vi "fpga_Filter Constant.vi"() -> (0 "Total Delay":u8=109, 1 "Start":fxp<+/-,4,4>=1.0, 2 "LP2 delay":u8=13, 3 "LP1 delay":u8=3)   [LabVIEW 2011, in "NI_EP_PMU_FPGA.lvlib"]
uses:
  <vilib>/addons/Electrical Power/PMU/NI_EP_PMU_FPGA.lvlib
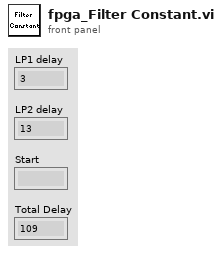
[diagram p1: front panel]
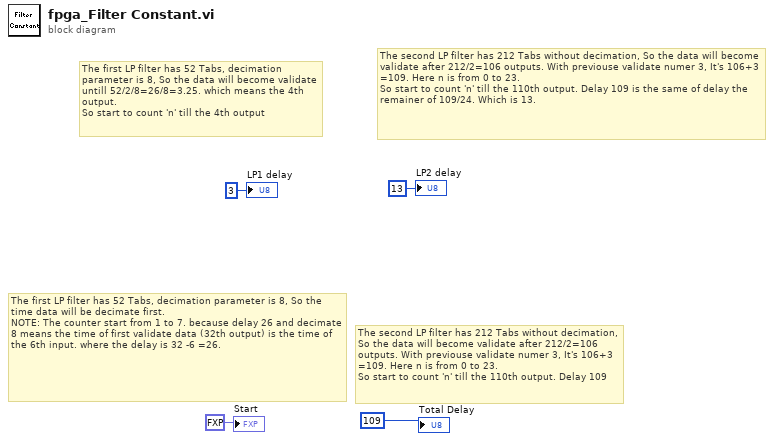
[diagram p0: block diagram]
diagram:
  # "The first LP filter has 52 Tabs, decimation parameter is 8, So the data will become validate untill 52/2/8=26/8=3.25. which means the 4th output.\nSo start to count 'n' till the 4th output"
  # "The second LP filter has 212 Tabs without decimation, So the data will become validate after 212/2=106 outputs. With previouse validate numer 3, It's 106+3 =109. Here n is from 0 to 23. \nSo start to count 'n' till the 110th output. Delay 109 is the same of delay the remainer of 109/24. Which is 13."
  # "The second LP filter has 212 Tabs without decimation, So the data will become validate after 212/2=106 outputs. With previouse validate numer 3, It's 106+3 =109. Here n is from 0 to 23. \nSo start to count 'n' till the 110th output. Delay 109"
  # "The first LP filter has 52 Tabs, decimation parameter is 8, So the time data will be decimate first.\nNOTE: The counter start from 1 to 7. because delay 26 and decimate 8 means the time of first validate data (32th output) is the time of the 6th input. where the delay is 32 -6 =26."
  "Start" <- fxp<+/-,4,4> 1.0 ("Start")
  "Total Delay" <- u8 109 ("Total Delay")
  "LP1 delay" <- u8 3 ("n-1[0..15]")
  "LP2 delay" <- u8 13 ("n-1[0..23]")
